vi "CMN_WriteCfgToMem.vi"(0 "Value":string, 1 "Ctrl type":string, 7 "Vi name":string, 9 "Ctrl name":string, 11 "error in":errorcluster) -> (15 "error out":errorcluster)   [LabVIEW 2016]
panel:
  in  "Types":string[](array[string])=["STR", "BOOL", "EXT", "DBL", "SGL", "I32", "I16", "I8", "U32", "U16", "U8", "FGEnum", "PATH", "U64", "I64"]
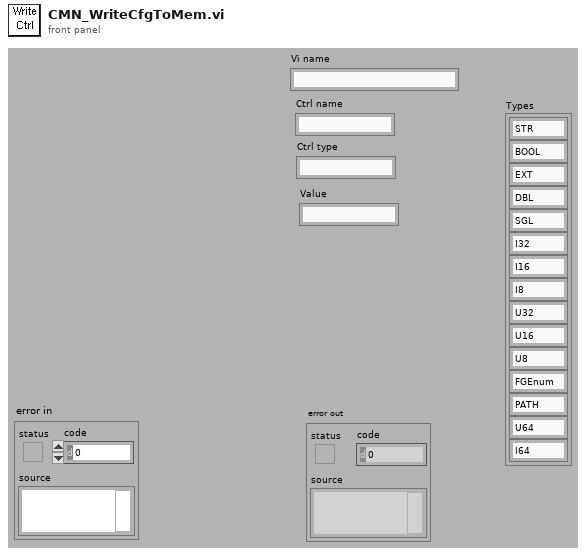
[diagram p1: front panel]
types:
  T1 = enum32{"Setup", "Settings", "Memory", "Utility", "Imaging", "Errors & Messages"}
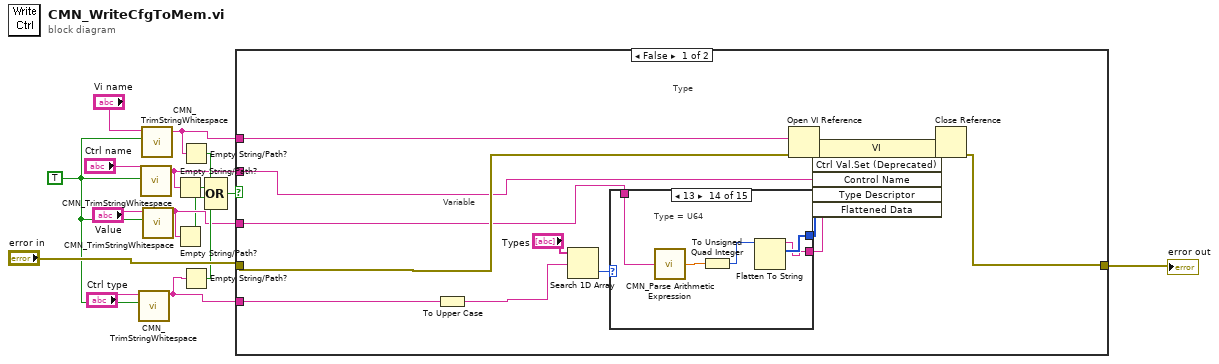
[diagram p0: block diagram]
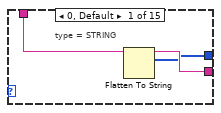
[diagram p2: hidden frame]
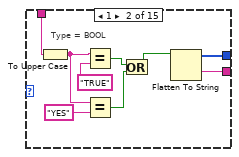
[diagram p3: hidden frame]
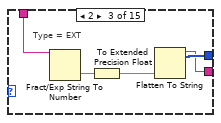
[diagram p4: hidden frame]
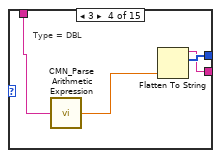
[diagram p5: hidden frame]
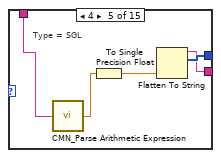
[diagram p6: hidden frame]
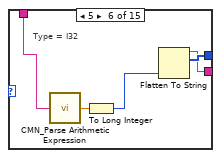
[diagram p7: hidden frame]
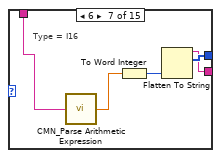
[diagram p8: hidden frame]
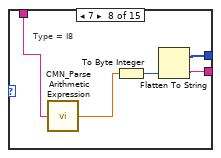
[diagram p9: hidden frame]
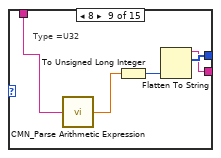
[diagram p10: hidden frame]
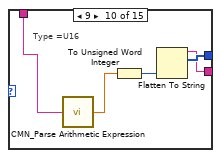
[diagram p11: hidden frame]
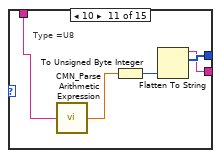
[diagram p12: hidden frame]
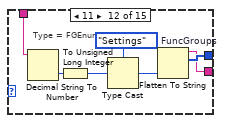
[diagram p13: hidden frame]
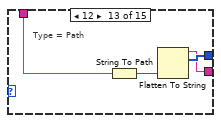
[diagram p14: hidden frame]
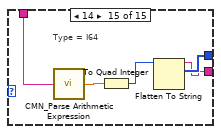
[diagram p15: hidden frame]
diagram:
  w10 = TRUE
  n1 = call "CMN_TrimStringWhitespace.vi"("Both Ends?(T)"=w10, "string"="Ctrl type") -> ("trimmed string"=w7:string)  [unwired: 8 out]
  n2 = call "CMN_TrimStringWhitespace.vi"("Both Ends?(T)"=w10, "string"="Ctrl name") -> ("trimmed string"=w3:string)  [unwired: 8 out]
  n3 = call "CMN_TrimStringWhitespace.vi"("Both Ends?(T)"=w10, "string"="Vi name") -> ("trimmed string"=w9:string)  [unwired: 8 out]
  n4 = call "CMN_TrimStringWhitespace.vi"("Both Ends?(T)"=w10, "string"="Value") -> ("trimmed string"=w5:string)  [unwired: 8 out]
  n5 = Empty String/Path?(string/path=w3) -> (empty?=w2:bool)
  n6 = Empty String/Path?(string/path=w5) -> (empty?=w4:bool)
  n7 = Empty String/Path?(string/path=w9) -> (empty?=w8:bool)
  n8 = Empty String/Path?(string/path=w7) -> (empty?=w6:bool)
  n9 = Compound Arithmetic op=OR(w8, w2, w4, w6) -> (w1:bool)
  n10 = case shown="False" w1 {
    tunnel: "error in" -> [w31 w109]
    tunnel: [w22 w109] -> w16
    tunnel: w9 -> [w21 _]
    tunnel: w3 -> [w20 _]
    tunnel: w5 -> [w19 _]
    tunnel: w7 -> [w18 _]
    frame False {
      # "Type"
      # "Variable"
      n11 = To Upper Case(1:w18) -> (0:w17:string)
      n12 = Search 1D Array(1D array="Types", element=w17) -> (index of element=w28:i32)  [unwired: 1 out]
      n13 = case shown="13" w28 {
        tunnel: [w33 w42 w47 w51 w55 w61 w65 w70 w75 w80 w85 w91 w97 w100 w105] -> w25
        tunnel: w19 -> [w34 w41 w46 w50 w54 w60 w64 w69 w74 w79 w84 w90 w95 w103 w108]
        tunnel: [w32 w43 w48 w52 w56 w62 w66 w71 w76 w81 w86 w92 w98 w101 w106] -> w26
        frame 0, Default {
          # "type = STRING"
          n14 = Flatten To String(anything=w34) -> (data string=w33:string, type string=w32:i16[])  [unwired: 1 in, 3 out]
        }
        frame 1 {
          # "Type = BOOL"
          n15 = To Upper Case(1:w41) -> (0:w37:string)
          n16 = Equal?(x=w37, y="TRUE") -> (x = y?=w38:bool)
          n17 = Equal?(x=w37, y="YES") -> (x = y?=w35:bool)
          n18 = Or(x=w38, y=w35) -> (x .or. y?=w39:bool)
          n19 = Flatten To String(anything=w39) -> (data string=w42:string, type string=w43:i16[])  [unwired: 1 in, 3 out]
        }
        frame 2 {
          # "Type = EXT"
          n20 = Fract/Exp String To Number(string=w46) -> (number=w45:dbl)  [unwired: 4 out]
          n21 = To Extended Precision Float(1:w45) -> (0:w44:ext)
          n22 = Flatten To String(anything=w44) -> (data string=w47:string, type string=w48:i16[])  [unwired: 1 in, 3 out]
        }
        frame 3 {
          # "Type = DBL"
          n23 = call "CMN_Parse Arithmetic Expression.vi"("Arithmetic Expression"=w50) -> ("Result"=w49:dbl)
          n24 = Flatten To String(anything=w49) -> (data string=w51:string, type string=w52:i16[])  [unwired: 1 in, 3 out]
        }
        frame 4 {
          # "Type = SGL"
          n25 = call "CMN_Parse Arithmetic Expression.vi"("Arithmetic Expression"=w54) -> ("Result"=w53:dbl)
          n26 = To Single Precision Float(number=w53) -> (single precision float=w57:sgl)
          n27 = Flatten To String(anything=w57) -> (data string=w55:string, type string=w56:i16[])  [unwired: 1 in, 3 out]
        }
        frame 5 {
          # "Type = I32"
          n28 = call "CMN_Parse Arithmetic Expression.vi"("Arithmetic Expression"=w60) -> ("Result"=w59:dbl)
          n29 = To Long Integer(number=w59) -> (32bit integer=w58:i32)
          n30 = Flatten To String(anything=w58) -> (data string=w61:string, type string=w62:i16[])  [unwired: 1 in, 3 out]
        }
        frame 6 {
          # "Type = I16"
          n31 = call "CMN_Parse Arithmetic Expression.vi"("Arithmetic Expression"=w64) -> ("Result"=w63:dbl)
          n32 = To Word Integer(number=w63) -> (16bit integer=w67:i16)
          n33 = Flatten To String(anything=w67) -> (data string=w65:string, type string=w66:i16[])  [unwired: 1 in, 3 out]
        }
        frame 7 {
          # "Type = I8"
          n34 = call "CMN_Parse Arithmetic Expression.vi"("Arithmetic Expression"=w69) -> ("Result"=w68:dbl)
          n35 = To Byte Integer(number=w68) -> (8bit integer=w72:i8)
          n36 = Flatten To String(anything=w72) -> (data string=w70:string, type string=w71:i16[])  [unwired: 1 in, 3 out]
        }
        frame 8 {
          # "Type =U32"
          n37 = call "CMN_Parse Arithmetic Expression.vi"("Arithmetic Expression"=w74) -> ("Result"=w73:dbl)
          n38 = To Unsigned Long Integer(number=w73) -> (unsigned 32bit integer=w77:u32)
          n39 = Flatten To String(anything=w77) -> (data string=w75:string, type string=w76:i16[])  [unwired: 1 in, 3 out]
        }
        frame 9 {
          # "Type =U16"
          n40 = call "CMN_Parse Arithmetic Expression.vi"("Arithmetic Expression"=w79) -> ("Result"=w78:dbl)
          n41 = To Unsigned Word Integer(number=w78) -> (unsigned 16bit integer=w82:u16)
          n42 = Flatten To String(anything=w82) -> (data string=w80:string, type string=w81:i16[])  [unwired: 1 in, 3 out]
        }
        frame 10 {
          # "Type =U8"
          n43 = call "CMN_Parse Arithmetic Expression.vi"("Arithmetic Expression"=w84) -> ("Result"=w83:dbl)
          n44 = To Unsigned Byte Integer(number=w83) -> (unsigned 8bit integer=w87:u8)
          n45 = Flatten To String(anything=w87) -> (data string=w85:string, type string=w86:i16[])  [unwired: 1 in, 3 out]
        }
        frame 11 {
          w88 = T1."Settings"  # FuncGroups
          # "Type = FGEnum"
          n46 = Decimal String To Number(string=w90) -> (number=w94:i32)  [unwired: 3 out]
          n47 = To Unsigned Long Integer(number=w94) -> (unsigned 32bit integer=w93:u32)
          n48 = Type Cast(type=w88, x=w93) -> (*(type *) &x=w89:T1)
          n49 = Flatten To String(anything=w89) -> (data string=w91:string, type string=w92:i16[])  [unwired: 1 in, 3 out]
        }
        frame 12 {
          # "Type = Path"
          n50 = String To Path(string=w95) -> (path=w96:path)
          n51 = Flatten To String(anything=w96) -> (data string=w97:string, type string=w98:i16[])  [unwired: 1 in, 3 out]
        }
        frame 13 {
          # "Type = U64"
          n52 = call "CMN_Parse Arithmetic Expression.vi"("Arithmetic Expression"=w103) -> ("Result"=w102:dbl)
          n53 = To Unsigned Quad Integer(1:w102) -> (0:w99:u64)
          n54 = Flatten To String(anything=w99) -> (data string=w100:string, type string=w101:i16[])  [unwired: 2 in, 2 out]
        }
        frame 14 {
          # "Type = I64"
          n55 = call "CMN_Parse Arithmetic Expression.vi"("Arithmetic Expression"=w108) -> ("Result"=w107:dbl)
          n56 = To Quad Integer(1:w107) -> (0:w104:i64)
          n57 = Flatten To String(anything=w104) -> (data string=w105:string, type string=w106:i16[])  [unwired: 2 in, 2 out]
        }
      }
      n58 = Open VI Reference(vi path=w21, error in (no error)=w31) -> (vi reference=w23:refnum<vi>, error out=w30:errorcluster)  [unwired: 4 out]
      n59 = invoke class="VI" method="Ctrl Val.Set (Deprecated)"(reference=w23, error in=w30, "Control Name"=w20, "Type Descriptor"=w26, "Flattened Data"=w25) -> (reference out=w29:refnum<vi>, error out=w24:errorcluster)  [unwired: 1 in, 4 out]
      n60 = Close Reference(reference=w29, error in (no error)=w24) -> (error out=w22:errorcluster)
    }
    frame True {
    }
  }
  "error out" <- w16
